vi "表格非空行数.vi"() -> (2 "行数":i32)   [LabVIEW 2015]
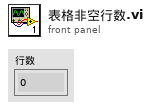
[diagram p1: front panel]
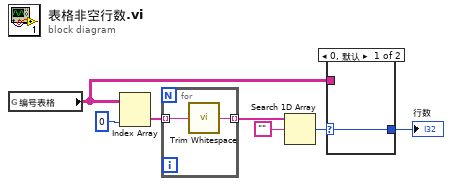
[diagram p0: block diagram]
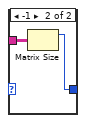
[diagram p2: hidden frame]
diagram:
  n1 = global read "全局.vi" "编号表格"() -> (w2:string[][])
  n2 = Index Array(array=w2, index (col)=0 ("禁用的索引 (列)")) -> (element=w6:string[])  [unwired: 1 in]
  n3 = for {
    tunnel: w6 -> [w9] mode=indexing
    tunnel: [w8] -> w4 mode=indexing
    n4 = call <vilib>:"Trim Whitespace.vi"("string"=w9) -> ("trimmed string"=w8:string)  [unwired: 1 in]
  }
  n5 = Search 1D Array(1D array=w4, element="") -> (index of element=w3:i32)  [unwired: 1 in]
  n6 = case shown="0, 默认" w3 {
    selector: w3 -> [w10 _]
    tunnel: w2 -> [_ w12]
    tunnel: [w10 w11] -> w1
    frame 0, Default {
    }
    frame -1 {
      n7 = Matrix Size(0:w12) -> (1:w11:i32)  [unwired: 1 out]
    }
  }
  "行数" <- w1
